vi "Row Col To Range.vi"(1 "Column":i32, 2 "Row":i32) -> (0 "Output String":string)   [LabVIEW 2020, in "NI_ReportGenerationToolkit.lvlib"]
doc: "Convert Row number and Column number into Excel Format of A1, A2,.. B1, B2.... and so on."
uses:
  <vilib>/addons/_office/NI_ReportGenerationToolkit.lvlib
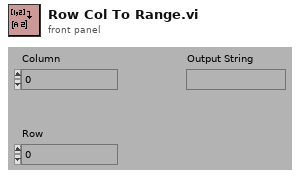
[diagram p1: front panel]
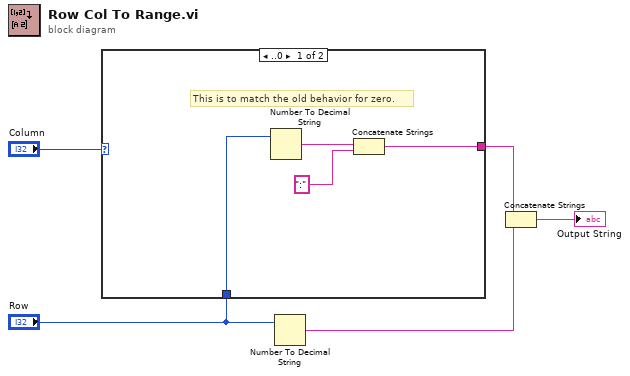
[diagram p0: block diagram]
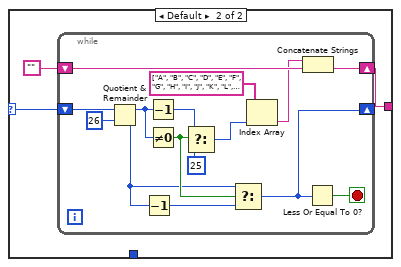
[diagram p2: hidden frame]
diagram:
  n1 = case shown="..0" "Column" {
    selector: "Column" -> [_ w10]
    tunnel: [w6 w11] -> w4
    tunnel: "Row" -> [w9 _]
    frame ..0 {
      # "This is to match the old behavior for zero."
      n2 = Number To Decimal String(number=w9) -> (decimal integer string=w8:string)  [unwired: 1 out]
      n3 = Concatenate Strings(w8, ":" ("string")) -> (w6:string)
    }
    frame Default {
      n4 = while {
        shift-right: [w25] -> w11
        shift-left: "" -> [w22]
        shift-right: [w15] -> _
        shift-left: w10 -> [w26]
        stop <- w24 stop-if-true
        n5 = Quotient & Remainder(x=w26, y=26) -> (x-y*floor(x/y)=w18:i32, floor(x/y)=w13:i32)
        n6 = Decrement(x=w13) -> (x-1=w16:i32)
        n7 = Decrement(x=w18) -> (x-1=w20:i32)
        n8 = Not Equal To 0?(x=w18) -> (x != 0?=w17:bool)
        n9 = Select(t=w20, s=w17, f=25) -> (s? t:f=w19:i32)
        n10 = Select(t=w13, s=w17, f=w16) -> (s? t:f=w15:i32)
        n11 = Index Array(array=string[] ["A", "B", "C", "D", "E", "F", "G", "H", "I", "J", "K", "L", "M", "N", "O", "P", "Q", "R", "S", "T", "U", "V", "W", "X", "Y", "Z"], index=w19) -> (element=w21:string)
        n12 = Concatenate Strings(w21, w22) -> (w25:string)
        n13 = Less Or Equal To 0?(x=w15) -> (x <= 0?=w24:bool)
      }
    }
  }
  n14 = Number To Decimal String(number="Row") -> (decimal integer string=w5:string)  [unwired: 1 out]
  n15 = Concatenate Strings(w4, w5) -> (→"Output String":string)
